vi "callback_func.vi"(4 "사용자 파라미터":variant, 5 "이벤트 데이터":cluster{"sender":refnum<k24>, "e":refnum<k24>}, 6 "컨트롤 참조":refnum<k24>, 7 "이벤트 일반 데이터":cluster{"이벤트 소스":i32, "이벤트 타입":u32, "타임스탬프":u32}) -> ()   [LabVIEW 2019]
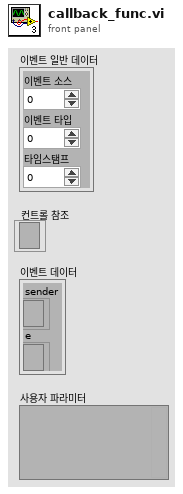
[diagram p1: front panel]
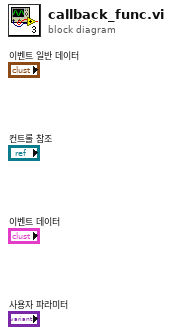
[diagram p0: block diagram]
diagram:
